vi "Mikrofon2.vi"() -> ()   [LabVIEW 2014]
uses:
  <vilib>/measure/maspectr.llb/FFT Power Spectrum and PSD for 1 Chan.vi
  <vilib>/measure/NI_MAPro.lvlib
panel:
  out "Frequency":dbl
  out "Maks frekvensen":dbl
  out "max index(es)":i32
  out "FFT power spectre":cluster{"f0":dbl, "df":dbl, "magnitude":dbl[]}(graph)
  out "magnitude":dbl[](array[numeric])
  out "df":dbl
  out "f0":dbl
  out "Soundsignal":waveform(dbl)(graph)
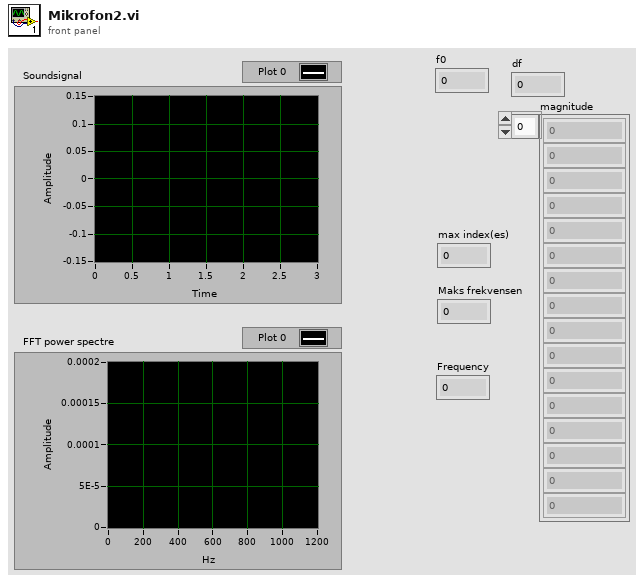
[diagram p1: front panel]
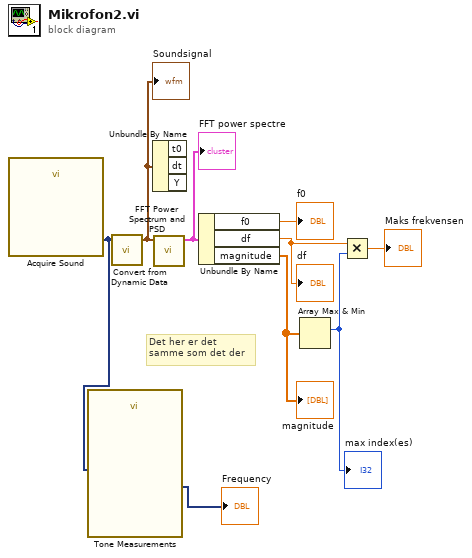
[diagram p0: block diagram]
diagram:
  # "Det her er det \nsamme som det der"
  n1 = call "Acquire Sound"() -> ("Data"=w2:dynamicdata)  [unwired: 18 in, 1 out]
  n2 = call "Tone Measurements"("Signals"=w2) -> ("Frequency"=→"Frequency":dynamicdata)  [unwired: 9 in, 1 out]
  n3 = call "Convert from Dynamic Data"("Dynamic Data Type"=w2) -> ("Waveform"=w9:waveform(dbl))  [unwired: 3 in]
  "Soundsignal" <- w9
  n4 = Unbundle By Name(w9) -> ()  [unwired: 3 out]
  n5 = call-poly <vilib>:"FFT Power Spectrum and PSD.vi"("time signal"=w9) -> ("Power Spectrum / PSD"=w7:cluster{"f0":dbl, "df":dbl, "magnitude":dbl[]})  [unwired: 7 in, 3 out]
  "FFT power spectre" <- w7
  n6 = Unbundle By Name(w7) -> ("f0"=→"f0":dbl, "df"=w5:dbl, "magnitude"=w6:dbl[])
  "df" <- w5
  "magnitude" <- w6
  n7 = Array Max & Min(array=w6) -> (max index (indices)=w4:i32)  [unwired: 3 out]
  "max index(es)" <- w4
  n8 = Multiply(x=w5, y=w4) -> (x*y=→"Maks frekvensen":dbl)
